vi "intake-shooter.vi"() -> ()   [LabVIEW 2023]
uses:
  ctrl defs/ctrl shooter speeds.ctl
  ctrl defs/ctrl intake speeds.ctl
  ctrl defs/ctrl INTAKE STATES.ctl
  ctrl defs/ctrl SHOOTER STATES.ctl
  <vilib>/Rock Robotics/WPI/MotorControl/WPI_MotorControlDeviceRef.ctl
  <vilib>/Rock Robotics/WPI/MotorControl/WPI_MotorControlType.ctl
  <vilib>/Rock Robotics/SystemInterfaces/DIO/FPGA_DIOPWMChannel.ctl
  <vilib>/Rock Robotics/WPI/PWM/WPI_PWMDeadband.ctl
  <vilib>/Rock Robotics/SystemInterfaces/DIO/FPGA_DIOChannel.ctl
  <vilib>/Rock Robotics/WPI/ThirdParty/REV Robotics/REVLib/Typedef/Spark MAX Control Type.ctl
  Global INIT.vi
  Global stack names.vi
  <vilib>/Rock Robotics/Network Tables/NT Read Boolean.vi
  <vilib>/Rock Robotics/Network Tables/NT Write String.vi
  <vilib>/Rock Robotics/Network Tables/NT Write Boolean.vi
panel:
  out "OVERIDE\nNOTE\nCHECK":bool
  in  "LOADER\nshoot\n%VBus":dbl
  in  "LOADER\nFeed Forward":dbl
  out "SHOOTER\ntarget %VBus":dbl=0.08
  out "Sensor Velocity":dbl=417.1380920410156
  out "SHOOTER\ntarget rpm":dbl=454.08
  out "SHOOTER\nVelocity (rpm)":dbl=417.1380920410156
  in  "AUTO run\nINTAKE after\nSHOT":bool
  in  "WRITE to global":bool
  in  "reload global values":bool
  in  "LOADER speeds":T1={"forward"=0.85, "reverse"=-1.0} {"reverse" min=-1.0 max=-0.02 format="%.3f"; "forward" min=0.02 max=1.0 format="%.3f"}
  in  "LOADER max/min":T1={"forward"=1.0, "reverse"=-1.0} {"reverse" min=-1.0 max=-0.02 format="%.3f"; "forward" min=0.02 max=1.0 format="%.3f"}
  in  "INTAKE speeds":T1={"forward"=1.0, "reverse"=-1.0} {"reverse" min=-1.0 max=-0.02 format="%.3f"; "forward" min=0.02 max=1.0 format="%.3f"}
  in  "SHOOTER speeds":T2={"SPEAKER"=1.0, "AMP"=0.08} {"AMP" min=0.02 max=1.0 format="%.3f"; "SPEAKER" min=0.02 max=1.0 format="%.3f"}
  in  "milliseconds to wait\nREV LOADER":u32=500
  in  "delay after\nSHOOT\ncommit (ms)":u32=500
  in  "delay for\nSPIN UP (ms)":u32=250
  in  "DISABLE\nNOTE CHECK for\nSHOOTING":bool=TRUE
  out "LOOKING\nfor NOTE":bool
  out "note sensor":bool
  in  "SHOOT STATUS":string="STANDBY"
  out "max rpm\n- SHOOTER":dbl=5676.0
  out "FIRE!":bool
  in  "INTAKE STATUS":string="Standby"
  out "max rpm\n- INTAKE":dbl=1419.0
  out "NOTE is\nloaded":bool
  out "run reverse":bool
  out "run intake":bool
  out "run? is\nACTIVE":bool
  in  "milliseconds to wait\nIN REVERSE":u32=1000
  in  "milliseconds to wait\nafter NOTE trigger":u32=100
  out "EXT FLAP":bool
  out "AMP OPT":bool
  in  "REVS to\nRETRACT":dbl=0.75 format="%#_13g"
  out "max rpm\n- LOADER":dbl=2750.0
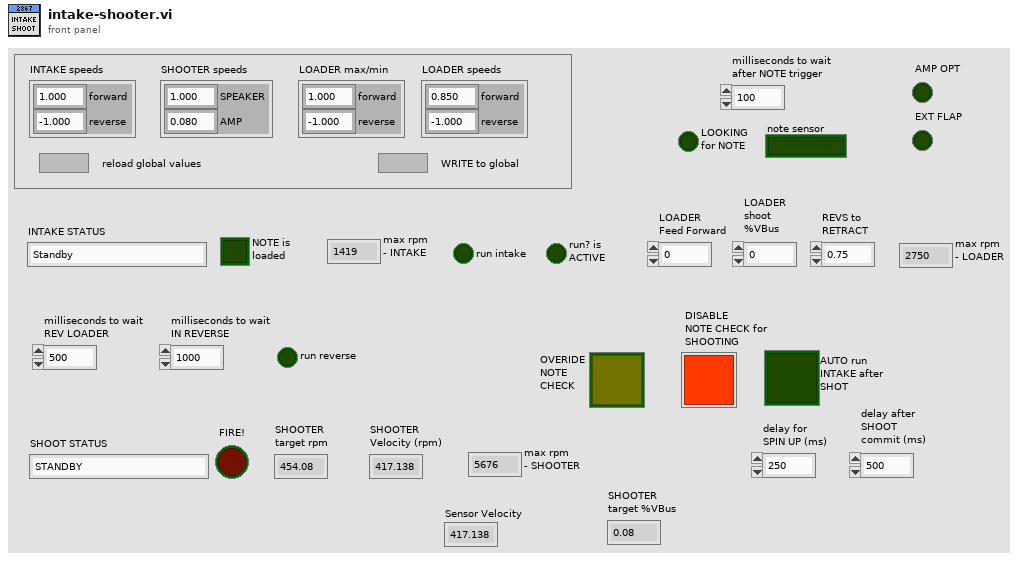
[diagram p1: front panel]
types:
  T1 = typedef "ctrl intake speeds.ctl" = cluster{"forward":dbl, "reverse":dbl}
  T2 = typedef "ctrl shooter speeds.ctl" = cluster{"SPEAKER":dbl, "AMP":dbl}
  T3 = typedef "ctrl SHOOTER STATES.ctl" = enum16{"STANDBY", "RETRACT NOTE", "SPIN-UP", "SHOOT", "RESET"}
  T4 = typedef "ctrl INTAKE STATES.ctl" = enum16{"STANDBY", "START INTAKES", "WATCH for NOTE", "SHUT DOWN", "REVERSE"}
  T5 = typedef "WPI_MotorControlDeviceRef.ctl" = cluster{"DeviceStatus":errorcluster, "Type":T6, "PWM":cluster{"PWM Channel":T7, "DeadBand":T8}, "CAN":cluster{"Device Number":u8, "SetOutput VI Ref":variant, "GetOutput VI Ref":variant, "Enable VI Ref":variant, "Disable VI Ref":variant, "Data":variant}, "Invert":bool, "DIO PWM":cluster{"PWM \"Enable\" Channel":T7, "DIOChannel":T9, "PWM Rate":dbl}}
  T6 = typedef "WPI_MotorControlType.ctl" = enum16{"PWM", "CAN", "DIO PWM"}
  T7 = typedef "FPGA_DIOPWMChannel.ctl" = enum8{"PWM 0", "PWM 1", "PWM 2", "PWM 3", "PWM 4", "PWM 5", "PWM 6", "PWM 7", "PWM 8", "PWM 9", "PWM MXP 0", "PWM MXP 1", "PWM MXP 2", "PWM MXP 3", "PWM MXP 4", "PWM MXP 5", "PWM MXP 6", "PWM MXP 7", "PWM MXP 8", "PWM MXP 9", "Invalid"}
  T8 = typedef "WPI_PWMDeadband.ctl" = cluster{"Name":string, "maxPositivePwm":i32, "minPositivePwm":i32, "centerPwm":i32, "maxNegativePwm":i32, "minNegativePwm":i32, "angularRange":u16}
  T9 = typedef "FPGA_DIOChannel.ctl" = enum8{"DIO 0", "DIO 1", "DIO 2", "DIO 3", "DIO 4", "DIO 5", "DIO 6", "DIO 7", "DIO 8", "DIO 9", "DIO MXP 0", "DIO MXP 1", "DIO MXP 2", "DIO MXP 3", "DIO MXP 4", "DIO MXP 5", "DIO MXP 6", "DIO MXP 7", "DIO MXP 8", "DIO MXP 9", "DIO MXP 10", "DIO MXP 11", "DIO MXP 12", "DIO MXP 13", "DIO MXP 14", "DIO MXP 15", "SPI Port CS1", "SPI Port CS2", "SPI Port CS3", "SPI Port MISO", "SPI Port MOSI", "Invalid"}
  T10 = cluster{"INTAKE ref":T5, "LOADER ref":T5, "SHOOTER ref":T5}
  T11 = typedef "ctrl DIO.ctl" = cluster{"description":string, "Installed?":bool, "DIOChannel":T9, "refnum name":string}
  T12 = typedef "ctrl swerve motor.ctl" = cluster{"description":string, "MOTOR SELECT":T13, "Installed?":bool, "CAN ID":u8, "refnum name":string, "Invert":bool, "Idle Mode":T14, "Current limiting":T15, "MOTOR PIDF coefficients":T16, "gear ratio":dbl}
  T13 = typedef "ctrl MOTOR SELECT.ctl" = i16
  T14 = typedef "Spark MAX Idle Mode.ctl" = enum16{"Coast", "Brake"}
  T15 = typedef "ctrl Spark MAX current limiting.ctl" = cluster{"Linearized":bool, "Free Speed (A)":dbl, "Primay (A)":dbl, "Limit RPM (0)":u32}
  T16 = typedef "ctrl motor PIDF coefficients.ctl" = cluster{"PIDF":cluster{"P Gain":dbl, "I Gain":dbl, "D Gain":dbl, "F Gain":dbl, "I Zone":dbl, "Min Output":dbl, "Max Output":dbl}, "Smart Motion":T17}
  T17 = typedef "Spark MAX Smart Motion Parameters.ctl" = cluster{"Max Velocity":dbl, "Max Acceleration":dbl, "Minimum Velocity Output":dbl, "Allowed Closed Loop Error":dbl}
  T18 = typedef "WPI_DigitalInputDevRef.ctl" = cluster{"DevStatus":errorcluster, "DIO Channel":T9}
  T19 = typedef "ctrl stack - INTAKE SHOOTER.ctl" = cluster{"INTAKE STATE":string, "RUN INTAKE?":string, "RUN REVERSE?":string, "NOTE LOADED?":string, "SHOOTER STATE":string, "SHOOTER FIRE?":string, "SHOOT AMP?":string, "EXTEND FLAP?":string, "LOOKING for NOTE":string, "OVERIDE NOTE CHECK":string}
  T20 = typedef "Spark MAX Control Type.ctl" = enum16{"Percent VBus", "Voltage", "Velocity", "Position", "Smart Motion", "Current", "Smart Velocity"}
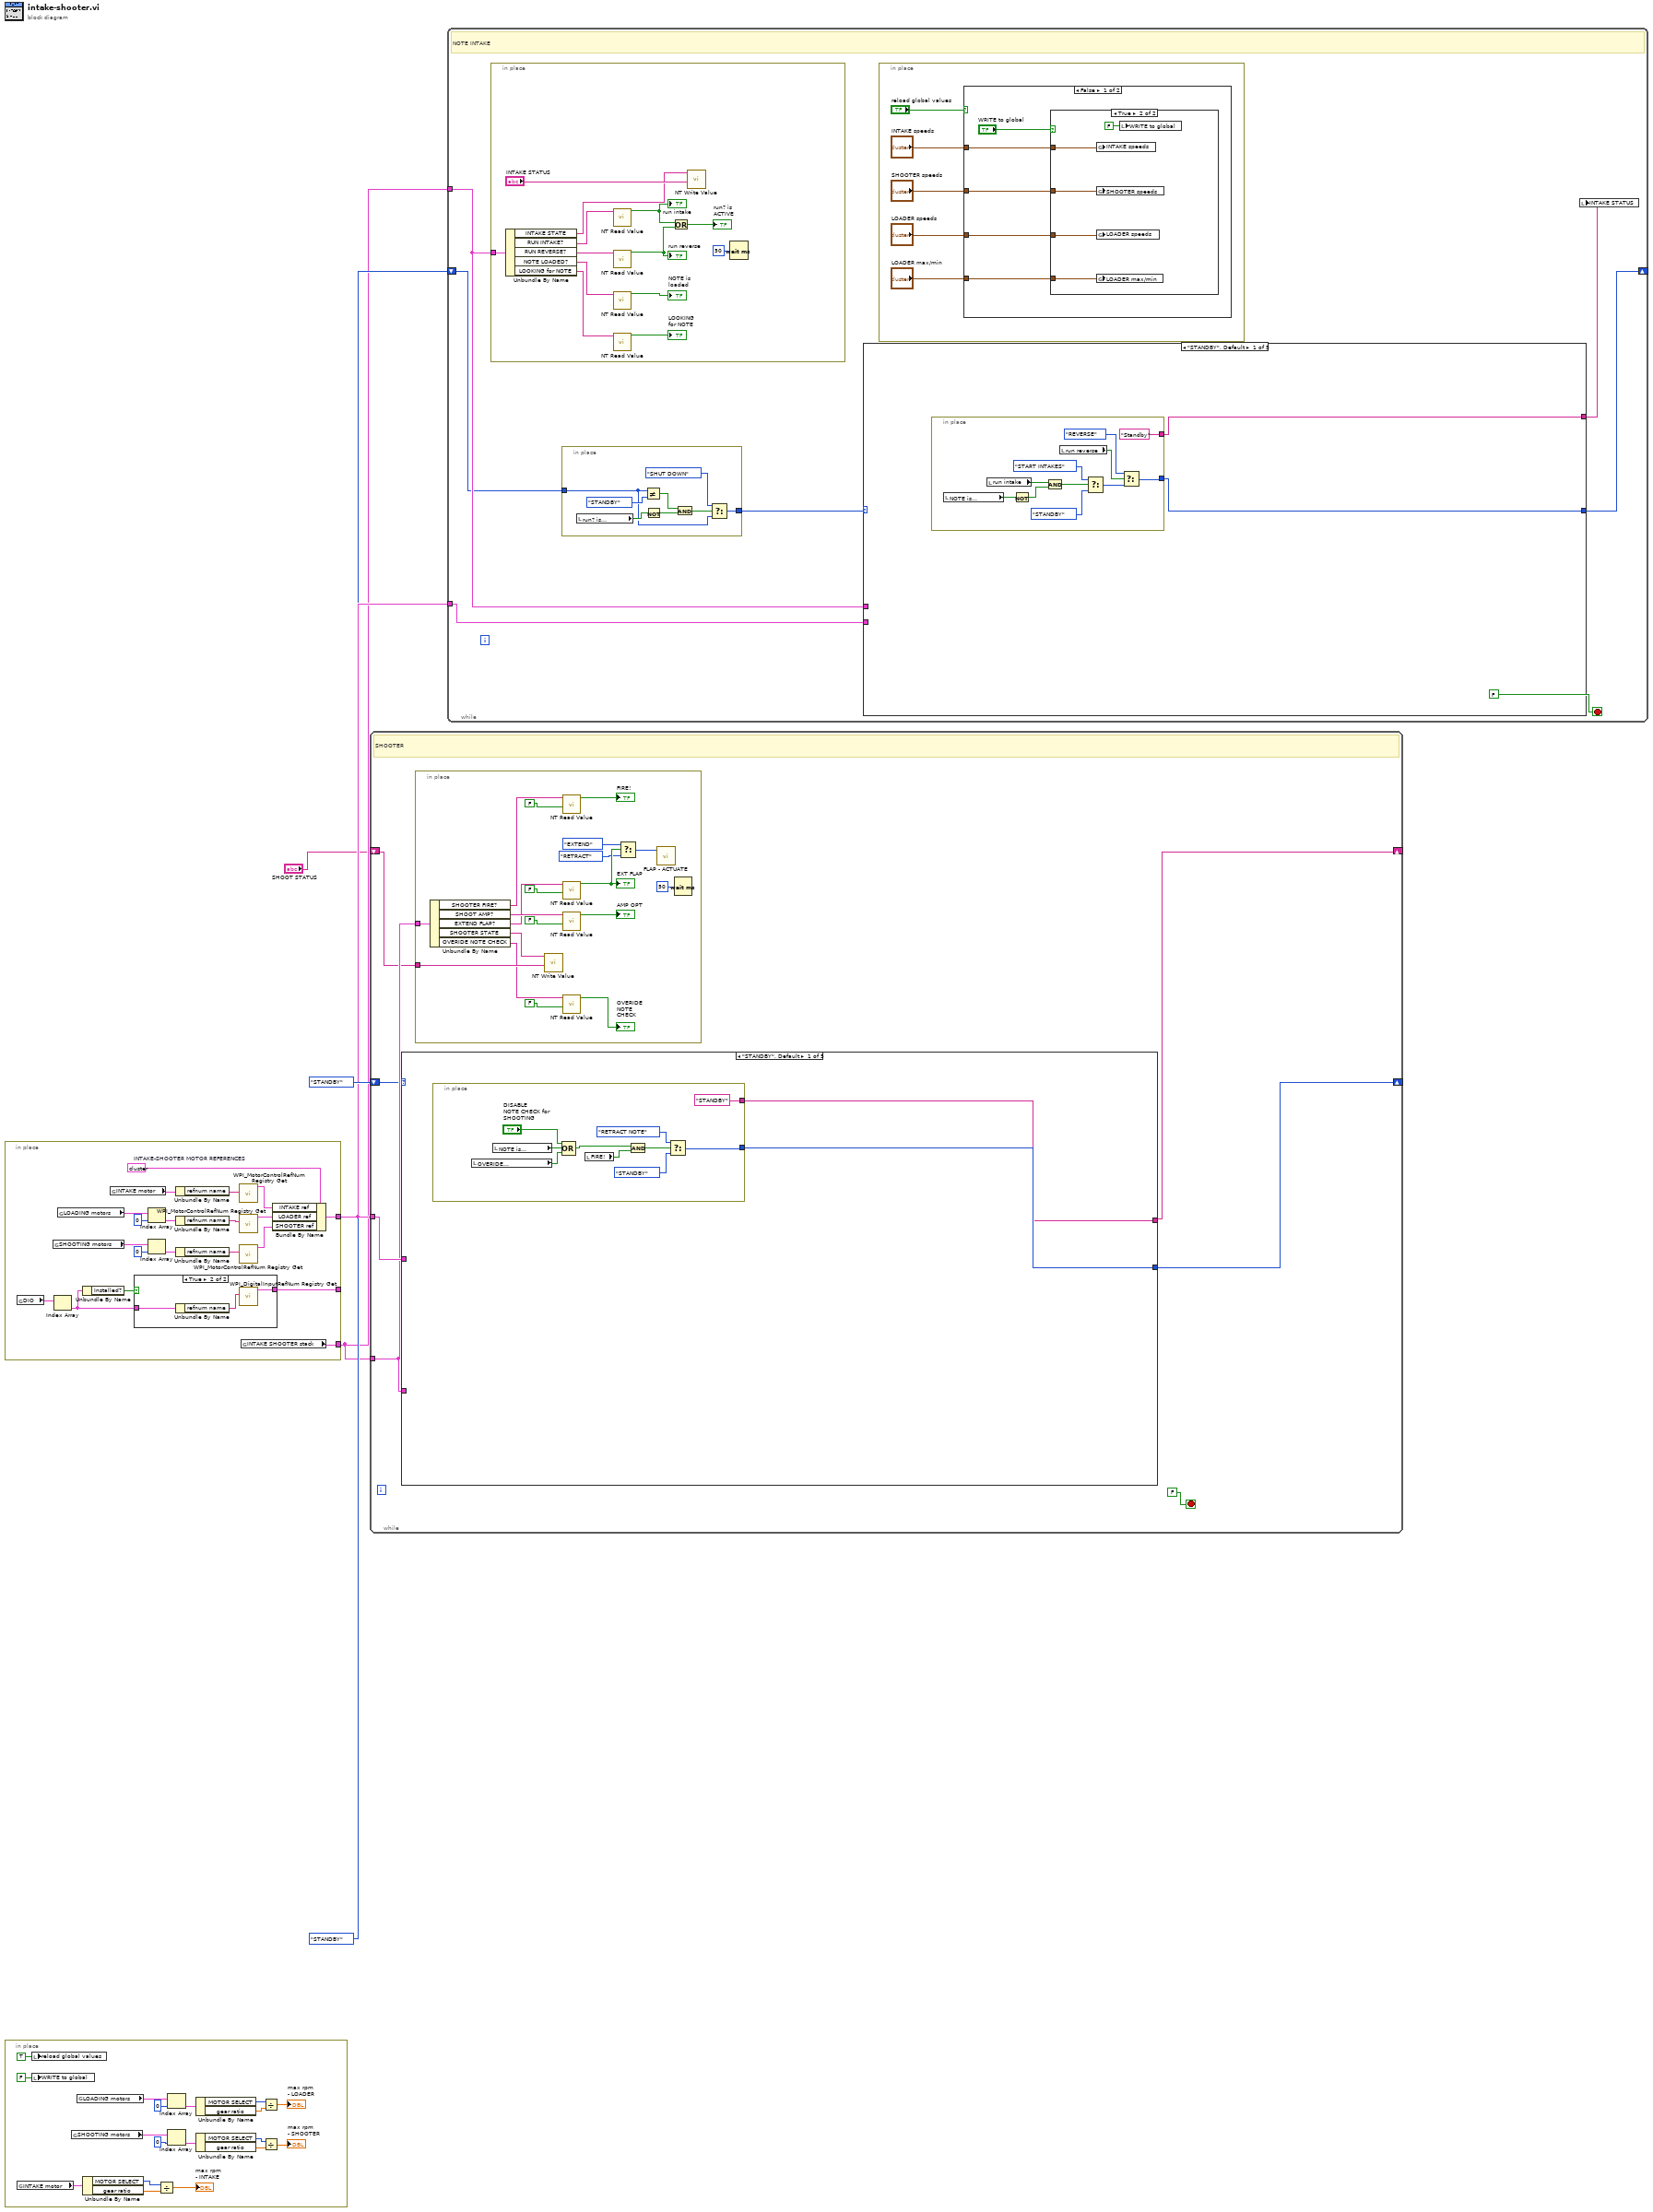
[diagram p0: block diagram]
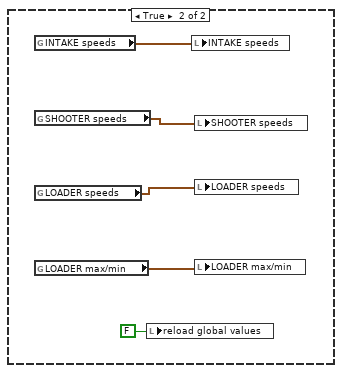
[diagram p3: hidden frame]
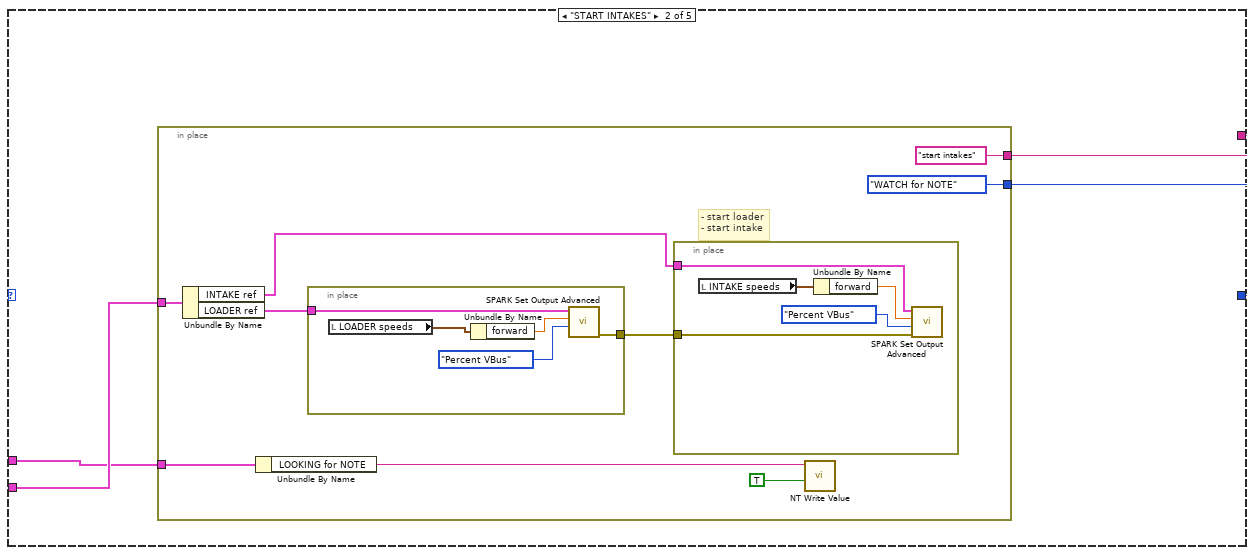
[diagram p4: hidden frame]
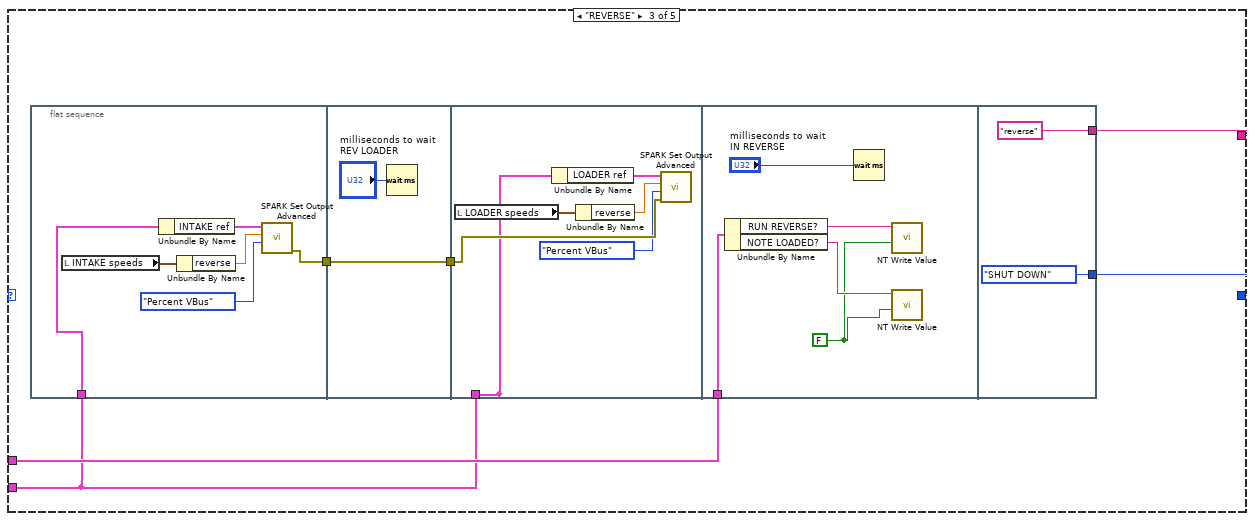
[diagram p5: hidden frame]
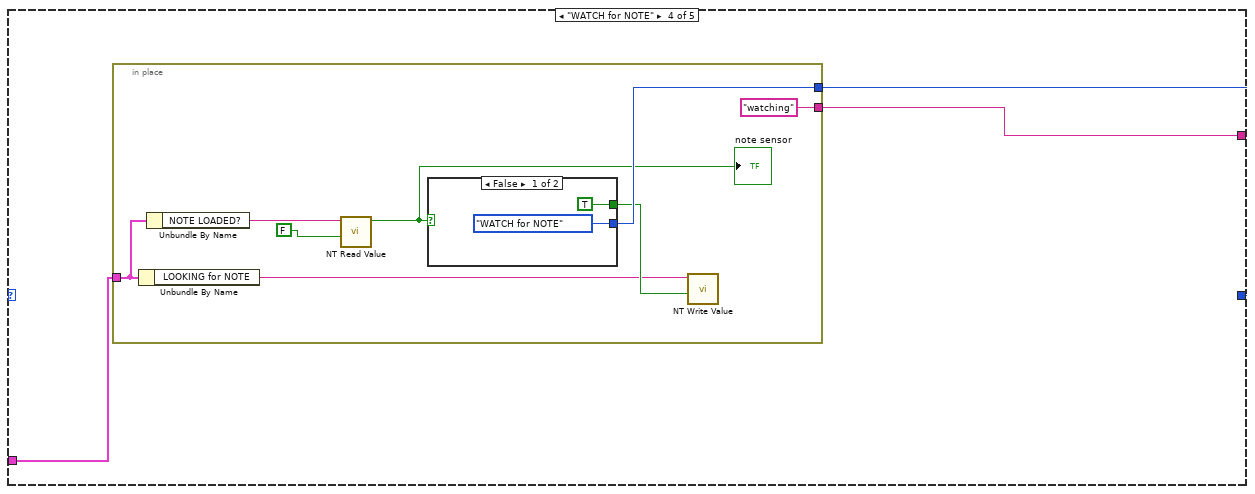
[diagram p6: hidden frame]
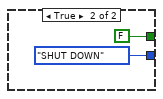
[diagram p7: hidden frame]
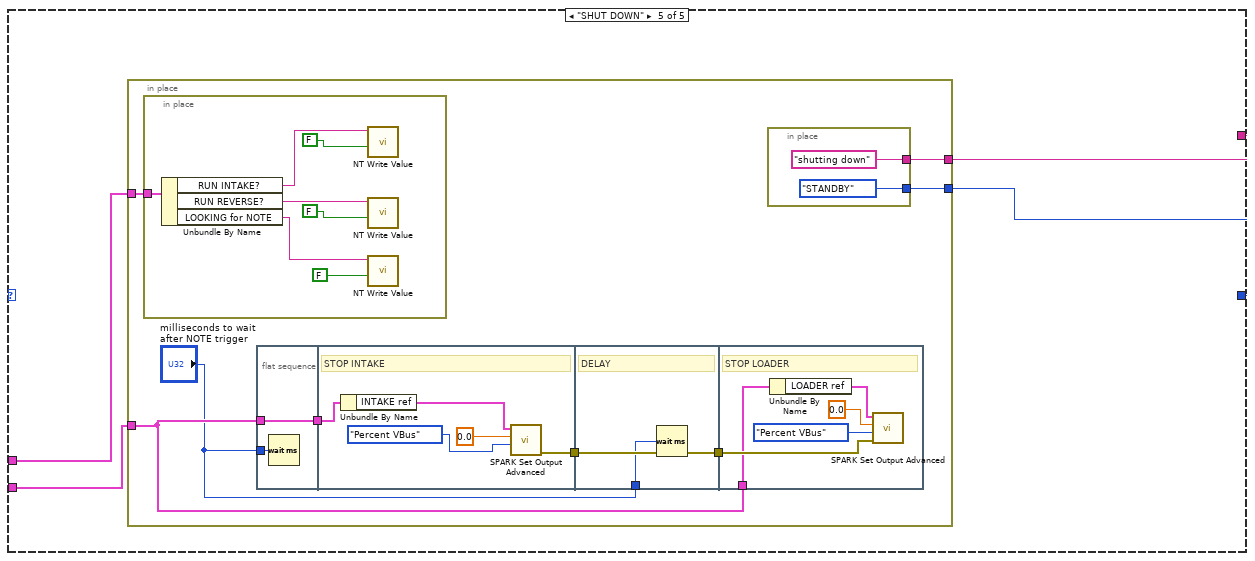
[diagram p8: hidden frame]
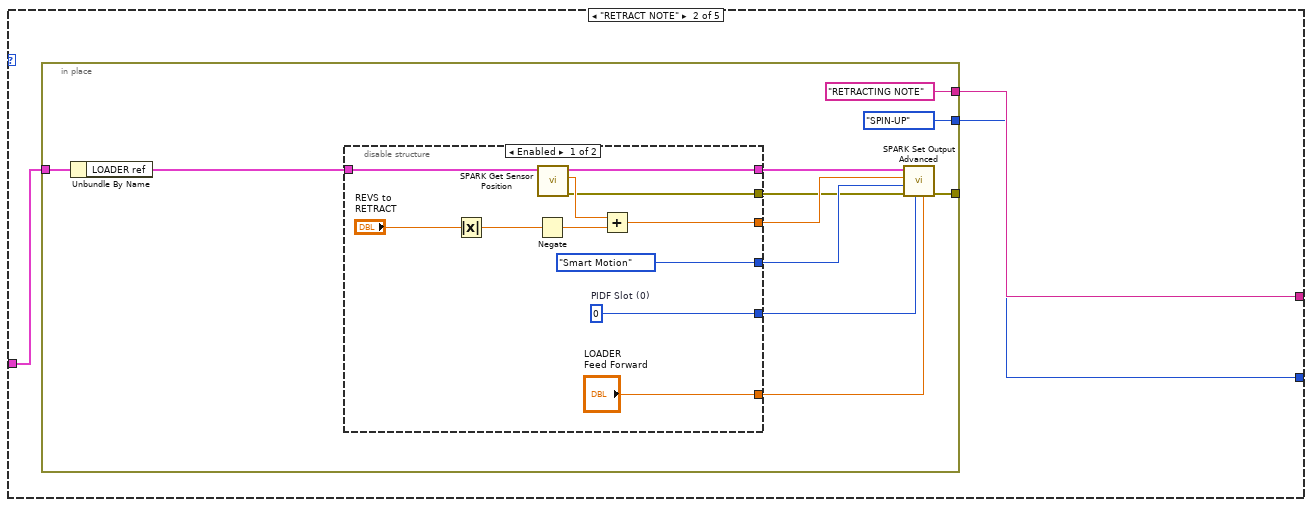
[diagram p9: hidden frame]
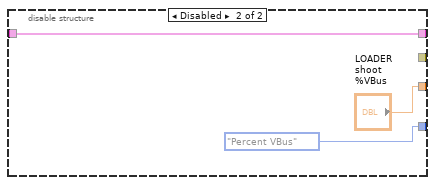
[diagram p10: hidden frame]
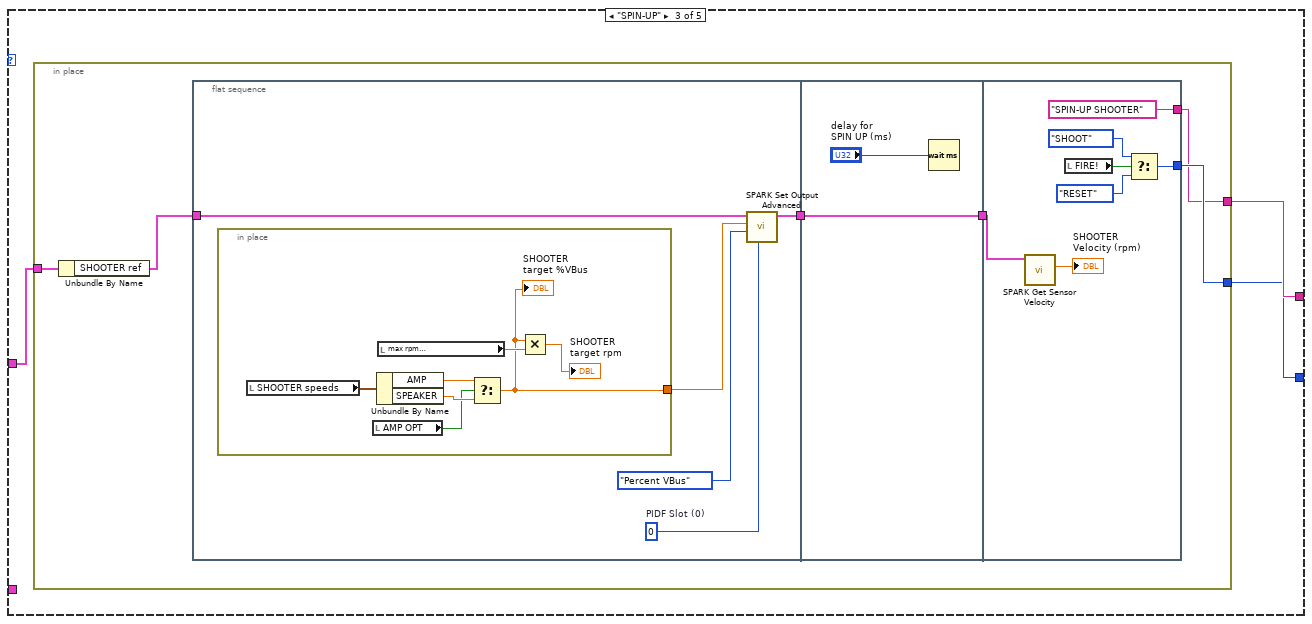
[diagram p11: hidden frame]
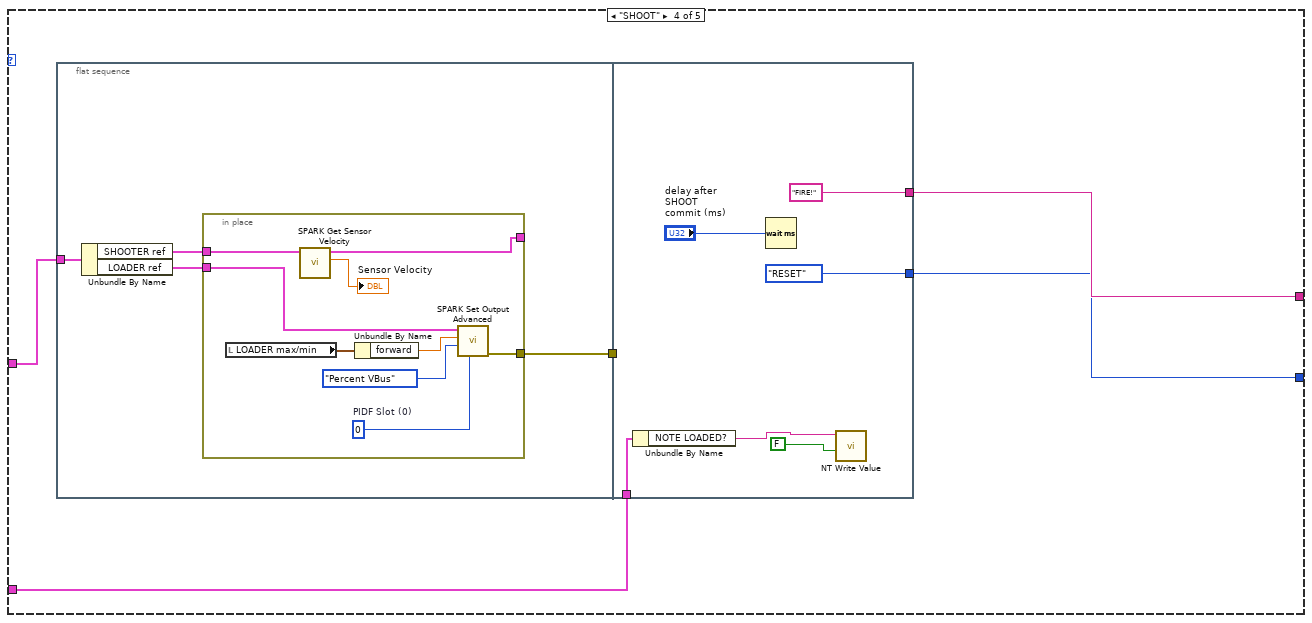
[diagram p12: hidden frame]
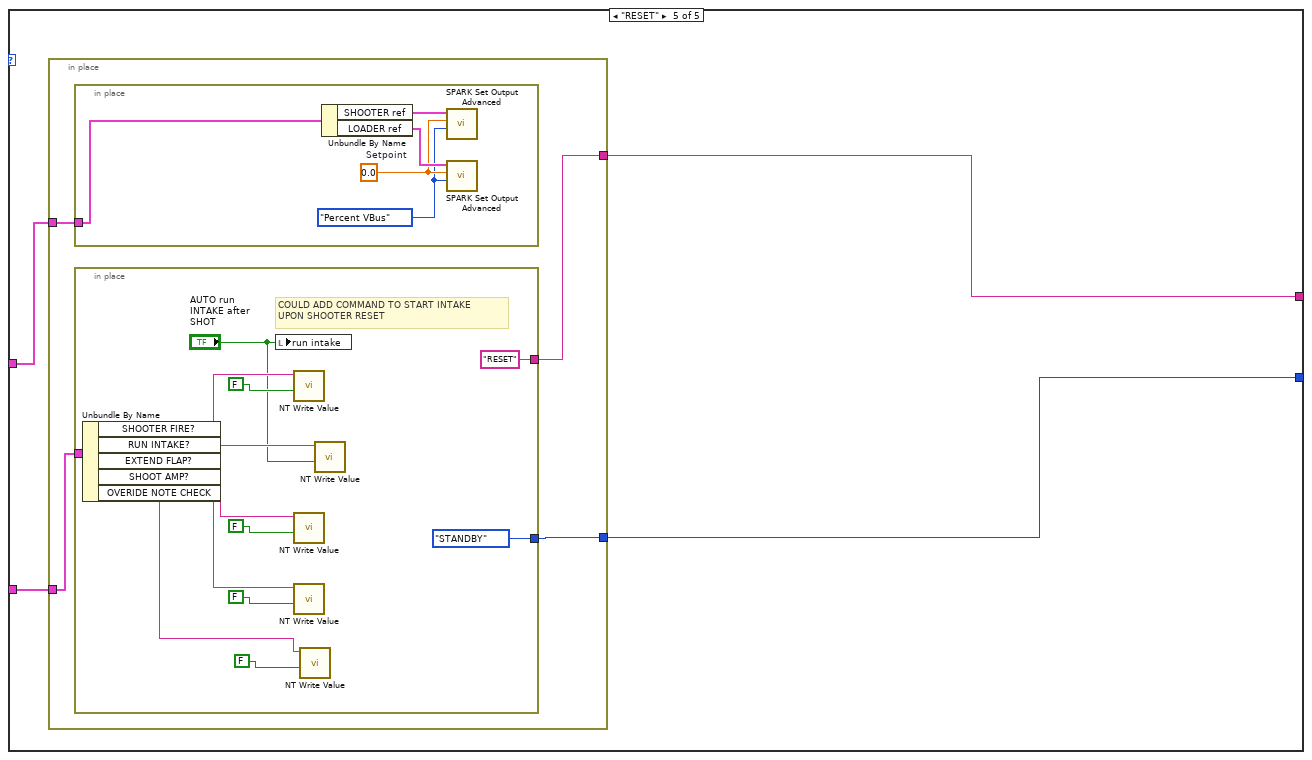
[diagram p13: hidden frame]
diagram:
  n1 = in-place {
    in-place-border: [w22] -> _
    in-place-border: [w7] -> w4
    in-place-border: [w6] -> w2
    w11 = T10 {"INTAKE ref"={"DeviceStatus"={"status"=FALSE, "code"=0, "source"=""}, "Type"=enum."PWM", "PWM"={"PWM Channel"=enum."Invalid", "DeadBand"={"Name"="", "maxPositivePwm"=0, "minPositivePwm"=0, "centerPwm"=0, "maxNegativePwm"=0, "minNegativePwm"=0, "angularRange"=0}}, "CAN"={"Device Number"=0, "SetOutput VI Ref"=variant(refnum<vi> refnum), "GetOutput VI Ref"=variant(refnum<vi> refnum), "Enable VI Ref"=variant(refnum<vi> refnum), "Disable VI Ref"=variant(refnum<vi> refnum), "Data"=variant}, "Invert"=FALSE, "DIO PWM"={"PWM \"Enable\" Channel"=enum."Invalid", "DIOChannel"=enum."Invalid", "PWM Rate"=0.0}}, "LOADER ref"={"DeviceStatus"={"status"=FALSE, "code"=0, "source"=""}, "Type"=enum."PWM", "PWM"={"PWM Channel"=enum."Invalid", "DeadBand"={"Name"="", "maxPositivePwm"=0, "minPositivePwm"=0, "centerPwm"=0, "maxNegativePwm"=0, "minNegativePwm"=0, "angularRange"=0}}, "CAN"={"Device Number"=0, "SetOutput VI Ref"=variant(refnum<vi> refnum), "GetOutput VI Ref"=variant(refnum<vi> refnum), "Enable VI Ref"=variant(refnum<vi> refnum), "Disable VI Ref"=variant(refnum<vi> refnum), "Data"=variant}, "Invert"=FALSE, "DIO PWM"={"PWM \"Enable\" Channel"=enum."Invalid", "DIOChannel"=enum."Invalid", "PWM Rate"=0.0}}, "SHOOTER ref"={"DeviceStatus"={"status"=FALSE, "code"=0, "source"=""}, "Type"=enum."PWM", "PWM"={"PWM Channel"=enum."Invalid", "DeadBand"={"Name"="", "maxPositivePwm"=0, "minPositivePwm"=0, "centerPwm"=0, "maxNegativePwm"=0, "minNegativePwm"=0, "angularRange"=0}}, "CAN"={"Device Number"=0, "SetOutput VI Ref"=variant(refnum<vi> refnum), "GetOutput VI Ref"=variant(refnum<vi> refnum), "Enable VI Ref"=variant(refnum<vi> refnum), "Disable VI Ref"=variant(refnum<vi> refnum), "Data"=variant}, "Invert"=FALSE, "DIO PWM"={"PWM \"Enable\" Channel"=enum."Invalid", "DIOChannel"=enum."Invalid", "PWM Rate"=0.0}}}  # INTAKE-SHOOTER MOTOR REFERENCES
    n2 = global read "Global INIT.vi" "DIO"() -> (w25:T11[])
    n3 = global read "Global INIT.vi" "SHOOTING motors"() -> (w20:T12[])
    n4 = Index Array(array=w25) -> (element=w23:T11)  [unwired: 1 in]
    n5 = global read "Global INIT.vi" "LOADING motors"() -> (w21:T12[])
    n6 = Unbundle By Name(w23) -> ("Installed?"=w24:bool)
    n7 = global read "Global INIT.vi" "INTAKE motor"() -> (w13:T12)
    n8 = case shown="True" w24 {
      tunnel: [_ w28] -> w22
      tunnel: w23 -> [_ w27]
      frame False {
      }
      frame True {
        n9 = Unbundle By Name(w27) -> ("refnum name"=w26:string)
        n10 = call <vilib>:"WPI_DigitalInputRefNum Registry Get.vi"("refnum name"=w26) -> ("DigitalInputDevRef"=w28:T18)  [unwired: 9 in, 1 out]
      }
    }
    n11 = Index Array(array=w21, index=0) -> (element=w17:T12)
    n12 = Index Array(array=w20, index=0) -> (element=w15:T12)
    n13 = Unbundle By Name(w13) -> ("refnum name"=w12:string)
    n14 = Unbundle By Name(w17) -> ("refnum name"=w16:string)
    n15 = Unbundle By Name(w15) -> ("refnum name"=w14:string)
    n16 = call <vilib>:"WPI_MotorControlRefNum Registry Get.vi"("refnum name"=w12) -> ("MotorControlDevRef"=w8:T5)  [unwired: 9 in, 1 out]
    n17 = call <vilib>:"WPI_MotorControlRefNum Registry Get.vi"("refnum name"=w16) -> ("MotorControlDevRef"=w9:T5)  [unwired: 9 in, 1 out]
    n18 = call <vilib>:"WPI_MotorControlRefNum Registry Get.vi"("refnum name"=w14) -> ("MotorControlDevRef"=w10:T5)  [unwired: 9 in, 1 out]
    n19 = global read "Global stack names.vi" "INTAKE SHOOTER stack"() -> (w6:T19)
    n20 = Bundle By Name(cluster=w11, "INTAKE ref"=w8, "LOADER ref"=w9, "SHOOTER ref"=w10) -> (w7:T10)
  }
  n21 = in-place {
    n22 = global read "Global INIT.vi" "INTAKE motor"() -> (w31:T12)
    n23 = local write "reload global values"(TRUE ("reload global values")) -> ()
    n24 = local write "WRITE to global"(FALSE ("WRITE to global")) -> ()
    n25 = global read "Global INIT.vi" "SHOOTING motors"() -> (w38:T12[])
    n26 = global read "Global INIT.vi" "LOADING motors"() -> (w43:T12[])
    n27 = Unbundle By Name(w31) -> ("MOTOR SELECT"=w33:T13, "gear ratio"=w32:dbl)
    n28 = Divide(x=w33, y=w32) -> (x/y=→"max rpm\n- INTAKE":dbl)
    n29 = Index Array(array=w43, index=0) -> (element=w41:T12)
    n30 = Index Array(array=w38, index=0) -> (element=w36:T12)
    n31 = Unbundle By Name(w41) -> ("MOTOR SELECT"=w40:T13, "gear ratio"=w39:dbl)
    n32 = Unbundle By Name(w36) -> ("MOTOR SELECT"=w35:T13, "gear ratio"=w34:dbl)
    n33 = Divide(x=w40, y=w39) -> (x/y=→"max rpm\n- LOADER":dbl)
    n34 = Divide(x=w35, y=w34) -> (x/y=→"max rpm\n- SHOOTER":dbl)
  }
  n35 = while {
    tunnel: w4 -> [w52]
    shift-right: [w53] -> _
    shift-left: ctrl_SHOOTER_STATES."STANDBY" -> [w49]
    tunnel: w2 -> [w50]
    shift-right: [w47] -> _
    shift-left: "SHOOT STATUS" -> [w48]
    stop <- FALSE stop-if-true
    # "SHOOTER"
    n36 = case shown="\"STANDBY\", Default" w49 {
      tunnel: [w55 w67 w94 w126 w149] -> w53
      tunnel: w52 -> [_ w66 w96 w128 w151]
      tunnel: [w54 w68 w95 w127 w150] -> w47
      tunnel: w50 -> [_ _ _ w124 w148]
      frame "STANDBY", Default {
        n37 = in-place {
          in-place-border: [w64] -> w55
          in-place-border: ["STANDBY" ("value")] -> w54
          n38 = local read "OVERIDE\nNOTE\nCHECK"() -> (w56:bool)
          n39 = local read "NOTE is\nloaded"() -> (w58:bool)
          n40 = Compound Arithmetic op=OR("DISABLE\nNOTE CHECK for\nSHOOTING", w58, w56) -> (w57:bool)
          n41 = local read "FIRE!"() -> (w62:bool)
          n42 = And(x=w57, y=w62) -> (x .and. y?=w63:bool)
          n43 = Select(t=ctrl_SHOOTER_STATES."RETRACT NOTE", s=w63, f=ctrl_SHOOTER_STATES."STANDBY") -> (s? t:f=w64:T3)
        }
      }
      frame "RETRACT NOTE" {
        n44 = in-place {
          in-place-border: ["RETRACTING NOTE" ("value")] -> w68
          in-place-border: [ctrl_SHOOTER_STATES."SPIN-UP"] -> w67
          in-place-border: [w73] -> _
          in-place-border: w66 -> [w72]
          n45 = Unbundle By Name(w72) -> ("LOADER ref"=w71:T5)
          n46 = disable-structure shown="Enabled" {
            disable-tunnel: [Spark_MAX_Control_Type."Smart Motion" ("Control Mode") Spark_MAX_Control_Type."Percent VBus" ("Control Mode")] -> w77
            disable-tunnel: [w89 _] -> w76
            disable-tunnel: [w88 w93] -> w75
            disable-tunnel: [w87 "LOADER\nshoot\n%VBus"] -> w74
            disable-tunnel: w71 -> [w85 w93]
            disable-tunnel: ["LOADER\nFeed Forward" _] -> w70
            disable-tunnel: [w80 _] -> w69
            frame Enabled {
              w89 = 0  # PIDF Slot (0)
              n47 = Absolute Value(x="REVS to\nRETRACT") -> (abs(x)=w83:dbl)
              n48 = Negate(x=w83) -> (-x=w82:dbl)
              n49 = call <vilib>:"SPARK Get Sensor Position.vi"("MotorControlDevRef in"=w85) -> ("error out"=w80:errorcluster, "Sensor Position"=w86:dbl, "MotorControlDevRef out"=w88:T5)  [unwired: 7 in, 1 out]
              n50 = Add(x=w86, y=w82) -> (x+y=w87:dbl)
            }
            frame Disabled {
            }
          }
          n51 = call <vilib>:"SPARK Set Output Advanced.vi"("Arbitrary Feed Forward (0)"=w70, "PIDF Slot (0)"=w76, "error in (no error)"=w69, "Control Mode"=w77, "Setpoint"=w74, "MotorControlDevRef"=w75) -> ("error out"=w73:errorcluster)  [unwired: 4 in, 1 out]
        }
      }
      frame "SPIN-UP" {
        n52 = in-place {
          in-place-border: w96 -> [w102]
          in-place-border: [w99] -> w95
          in-place-border: [w100] -> w94
          n53 = Unbundle By Name(w102) -> ("SHOOTER ref"=w101:T5)
          n54 = flat-sequence {
            tunnel: w101 -> [w107]
            tunnel: [w104] -> w98
            tunnel: w98 -> [w115]
            tunnel: [w115] -> w97
            tunnel: [w121] -> w100
            tunnel: ["SPIN-UP SHOOTER" ("value")] -> w99
            tunnel: w97 -> [w117]
            frame #0 {
              w105 = 0  # PIDF Slot (0)
              n55 = in-place {
                in-place-border: [w108] -> w103
                n56 = local read "SHOOTER speeds"() -> (w111:T2)
                n57 = local read "AMP OPT"() -> (w112:bool)
                n58 = Unbundle By Name(w111) -> ("AMP"=w113:dbl, "SPEAKER"=w114:dbl)
                n59 = local read "max rpm\n- SHOOTER"() -> (w109:dbl)
                n60 = Select(t=w113, s=w112, f=w114) -> (s? t:f=w108:dbl)
                "SHOOTER\ntarget %VBus" <- w108
                n61 = Multiply(x=w108, y=w109) -> (x*y=→"SHOOTER\ntarget rpm":dbl)
              }
              n62 = call <vilib>:"SPARK Set Output Advanced.vi"("PIDF Slot (0)"=w105, "Control Mode"=Spark_MAX_Control_Type."Percent VBus", "Setpoint"=w103, "MotorControlDevRef"=w107) -> ("MotorControlDevRef"=w104:T5)  [unwired: 6 in, 1 out]
            }
            frame #1 {
              n63 = Wait (ms)(milliseconds to wait="delay for\nSPIN UP (ms)") -> ()  [unwired: 1 out]
            }
            frame #2 {
              n64 = call <vilib>:"SPARK Get Sensor Velocity.vi"("MotorControlDevRef in"=w117) -> ("Sensor Velocity"=→"SHOOTER\nVelocity (rpm)":dbl)  [unwired: 7 in, 3 out]
              n65 = local read "FIRE!"() -> (w123:bool)
              n66 = Select(t=ctrl_SHOOTER_STATES."SHOOT", s=w123, f=ctrl_SHOOTER_STATES."RESET") -> (s? t:f=w121:T3)
            }
          }
        }
      }
      frame "SHOOT" {
        n67 = flat-sequence {
          tunnel: w128 -> [w132]
          tunnel: [w129] -> w125
          tunnel: ["FIRE!" ("value")] -> w127
          tunnel: [ctrl_SHOOTER_STATES."RESET"] -> w126
          tunnel: w125 -> [_]
          tunnel: w124 -> [w142]
          frame #0 {
            n68 = Unbundle By Name(w132) -> ("SHOOTER ref"=w130:T5, "LOADER ref"=w131:T5)
            n69 = in-place {
              in-place-border: w131 -> [w141]
              in-place-border: w130 -> [w136]
              in-place-border: [w135] -> _
              in-place-border: [w134] -> w129
              w140 = 0  # PIDF Slot (0)
              n70 = local read "LOADER max/min"() -> (w138:T1)
              n71 = call <vilib>:"SPARK Get Sensor Velocity.vi"("MotorControlDevRef in"=w136) -> ("Sensor Velocity"=→"Sensor Velocity":dbl, "MotorControlDevRef out"=w135:T5)  [unwired: 7 in, 2 out]
              n72 = Unbundle By Name(w138) -> ("forward"=w137:dbl)
              n73 = call <vilib>:"SPARK Set Output Advanced.vi"("PIDF Slot (0)"=w140, "Control Mode"=Spark_MAX_Control_Type."Percent VBus", "Setpoint"=w137, "MotorControlDevRef"=w141) -> ("error out"=w134:errorcluster)  [unwired: 6 in, 1 out]
            }
          }
          frame #1 {
            n74 = Unbundle By Name(w142) -> ("NOTE LOADED?"=w144:string)
            n75 = Wait (ms)(milliseconds to wait="delay after\nSHOOT\ncommit (ms)") -> ()  [unwired: 1 out]
            n76 = call-poly <vilib>:"NT Write Value.vi"("value"=FALSE, "name"=w144) -> ()  [unwired: 9 in, 1 out]
          }
        }
      }
      frame "RESET" {
        n77 = in-place {
          in-place-border: w151 -> [w155]
          in-place-border: [w152] -> w150
          in-place-border: [w153] -> w149
          in-place-border: w148 -> [w154]
          n78 = in-place {
            in-place-border: w155 -> [w158]
            w157 = 0.0  # Setpoint
            w156 = Spark_MAX_Control_Type."Percent VBus" ("Control Mode")
            n79 = Unbundle By Name(w158) -> ("SHOOTER ref"=w159:T5, "LOADER ref"=w160:T5)
            n80 = call <vilib>:"SPARK Set Output Advanced.vi"("Control Mode"=w156, "Setpoint"=w157, "MotorControlDevRef"=w159) -> ()  [unwired: 7 in, 2 out]
            n81 = call <vilib>:"SPARK Set Output Advanced.vi"("Control Mode"=w156, "Setpoint"=w157, "MotorControlDevRef"=w160) -> ()  [unwired: 7 in, 2 out]
          }
          n82 = in-place {
            in-place-border: w154 -> [w172]
            in-place-border: [ctrl_SHOOTER_STATES."STANDBY"] -> w153
            in-place-border: ["RESET" ("value")] -> w152
            # "COULD ADD COMMAND TO START INTAKE\nUPON SHOOTER RESET"
            n83 = Unbundle By Name(w172) -> ("SHOOTER FIRE?"=w171:string, "RUN INTAKE?"=w170:string, "EXTEND FLAP?"=w168:string, "SHOOT AMP?"=w165:string, "OVERIDE NOTE CHECK"=w161:string)
            n84 = local write "run intake"("AUTO run\nINTAKE after\nSHOT") -> ()
            n85 = call-poly <vilib>:"NT Write Value.vi"("value"=FALSE ("default value"), "name"=w171) -> ()  [unwired: 9 in, 1 out]
            n86 = call-poly <vilib>:"NT Write Value.vi"("value"=FALSE, "name"=w168) -> ()  [unwired: 9 in, 1 out]
            n87 = call-poly <vilib>:"NT Write Value.vi"("value"=FALSE, "name"=w165) -> ()  [unwired: 9 in, 1 out]
            n88 = call-poly <vilib>:"NT Write Value.vi"("value"=FALSE, "name"=w161) -> ()  [unwired: 9 in, 1 out]
            n89 = call-poly <vilib>:"NT Write Value.vi"("value"="AUTO run\nINTAKE after\nSHOT", "name"=w170) -> ()  [unwired: 9 in, 1 out]
          }
        }
      }
    }
    n90 = in-place {
      in-place-border: w50 -> [w191]
      in-place-border: w48 -> [w177]
      n91 = Unbundle By Name(w191) -> ("SHOOTER FIRE?"=w190:string, "SHOOT AMP?"=w188:string, "EXTEND FLAP?"=w185:string, "SHOOTER STATE"=w179:string, "OVERIDE NOTE CHECK"=w176:string)
      n92 = call-poly <vilib>:"NT Write Value.vi"("value"=w177, "name"=w179) -> ()  [unwired: 9 in, 1 out]
      n93 = call-poly <vilib>:"NT Read Value.vi"("default value"=FALSE, "name"=w190) -> ("value"=→"FIRE!":bool)  [unwired: 7 in, 2 out]
      n94 = call-poly <vilib>:"NT Read Value.vi"("default value"=FALSE, "name"=w185) -> ("value"=w182:bool)  [unwired: 7 in, 2 out]
      "EXT FLAP" <- w182
      n95 = call-poly <vilib>:"NT Read Value.vi"("default value"=FALSE, "name"=w188) -> ("value"=→"AMP OPT":bool)  [unwired: 7 in, 2 out]
      n96 = call-poly <vilib>:"NT Read Value.vi"("default value"=FALSE, "name"=w176) -> ("value"=→"OVERIDE\nNOTE\nCHECK":bool)  [unwired: 7 in, 2 out]
      n97 = Select(t=enum16{"EXTEND", "RETRACT"}."EXTEND" ("STATE"), s=w182, f=enum16{"EXTEND", "RETRACT"}."RETRACT" ("STATE")) -> (s? t:f=w184:enum16{"EXTEND", "RETRACT"})
      n98 = call "FLAP - ACTUATE.vi"("STATE"=w184) -> ()  [unwired: 10 in, 1 out]
      n99 = Wait (ms)(milliseconds to wait=u32 50) -> ()  [unwired: 1 out]
    }
  }
  n100 = while {
    shift-right: [w198] -> _
    shift-left: ctrl_INTAKE_STATES."STANDBY" ("INTAKE STATE") -> [w196]
    tunnel: w4 -> [w193]
    tunnel: w2 -> [w197]
    stop <- FALSE stop-if-true
    # "NOTE INTAKE"
    n101 = in-place {
      in-place-border: w197 -> [w349]
      n102 = Unbundle By Name(w349) -> ("INTAKE STATE"=w344:string, "RUN INTAKE?"=w351:string, "RUN REVERSE?"=w350:string, "NOTE LOADED?"=w352:string, "LOOKING for NOTE"=w341:string)
      n103 = call-poly <vilib>:"NT Read Value.vi"("name"=w351) -> ("value"=w348:bool)  [unwired: 8 in, 2 out]
      "run intake" <- w348
      n104 = call-poly <vilib>:"NT Read Value.vi"("name"=w350) -> ("value"=w347:bool)  [unwired: 8 in, 2 out]
      "run reverse" <- w347
      n105 = call-poly <vilib>:"NT Read Value.vi"("name"=w352) -> ("value"=→"NOTE is\nloaded":bool)  [unwired: 8 in, 2 out]
      n106 = call-poly <vilib>:"NT Read Value.vi"("name"=w341) -> ("value"=→"LOOKING\nfor NOTE":bool)  [unwired: 8 in, 2 out]
      n107 = Or(x=w348, y=w347) -> (x .or. y?=→"run? is\nACTIVE":bool)
      n108 = call-poly <vilib>:"NT Write Value.vi"("value"="INTAKE STATUS", "name"=w344) -> ()  [unwired: 9 in, 1 out]
      n109 = Wait (ms)(milliseconds to wait=u32 50) -> ()  [unwired: 1 out]
    }
    n110 = in-place {
      in-place-border: w196 -> [w220]
      in-place-border: [w223] -> w195
      n111 = local read "run? is\nACTIVE"() -> (w224:bool)
      n112 = Not Equal?(x=w220, y=ctrl_INTAKE_STATES."STANDBY" ("INTAKE STATE")) -> (x != y?=w227:bool)
      n113 = Not(x=w224) -> (.not. x?=w225:bool)
      n114 = And(x=w227, y=w225) -> (x .and. y?=w221:bool)
      n115 = Select(t=ctrl_INTAKE_STATES."SHUT DOWN" ("INTAKE STATE"), s=w221, f=w220) -> (s? t:f=w223:T4)
    }
    n116 = case shown="\"STANDBY\", Default" w195 {
      tunnel: [w229 w244 w268 w292 w309] -> w198
      tunnel: [w228 w243 w267 w293 w308] -> w194
      tunnel: w193 -> [_ w242 w264 _ w307]
      tunnel: w197 -> [_ w241 w269 w291 w306]
      frame "STANDBY", Default {
        n117 = in-place {
          in-place-border: [w235] -> w229
          in-place-border: ["Standby" ("value")] -> w228
          n118 = local read "NOTE is\nloaded"() -> (w232:bool)
          n119 = local read "run intake"() -> (w231:bool)
          n120 = Not(x=w232) -> (.not. x?=w238:bool)
          n121 = And(x=w231, y=w238) -> (x .and. y?=w239:bool)
          n122 = local read "run reverse"() -> (w233:bool)
          n123 = Select(t=ctrl_INTAKE_STATES."START INTAKES" ("INTAKE STATE 2"), s=w239, f=ctrl_INTAKE_STATES."STANDBY" ("INTAKE STATE 2")) -> (s? t:f=w236:T4)
          n124 = Select(t=ctrl_INTAKE_STATES."REVERSE" ("INTAKE STATE 2"), s=w233, f=w236) -> (s? t:f=w235:T4)
        }
      }
      frame "START INTAKES" {
        n125 = in-place {
          in-place-border: [ctrl_INTAKE_STATES."WATCH for NOTE" ("INTAKE STATE 2")] -> w244
          in-place-border: ["start intakes" ("value")] -> w243
          in-place-border: w242 -> [w251]
          in-place-border: w241 -> [w246]
          # "- start loader\n- start intake"
          n126 = Unbundle By Name(w251) -> ("INTAKE ref"=w250:T5, "LOADER ref"=w249:T5)
          n127 = Unbundle By Name(w246) -> ("LOOKING for NOTE"=w247:string)
          n128 = in-place {
            in-place-border: w249 -> [w258]
            in-place-border: [w256] -> w248
            n129 = local read "LOADER speeds"() -> (w254:T1)
            n130 = Unbundle By Name(w254) -> ("forward"=w255:dbl)
            n131 = call <vilib>:"SPARK Set Output Advanced.vi"("Control Mode"=Spark_MAX_Control_Type."Percent VBus", "Setpoint"=w255, "MotorControlDevRef"=w258) -> ("error out"=w256:errorcluster)  [unwired: 7 in, 1 out]
          }
          n132 = in-place {
            in-place-border: w250 -> [w263]
            in-place-border: w248 -> [w261]
            n133 = local read "INTAKE speeds"() -> (w260:T1)
            n134 = Unbundle By Name(w260) -> ("forward"=w259:dbl)
            n135 = call <vilib>:"SPARK Set Output Advanced.vi"("error in (no error)"=w261, "Control Mode"=Spark_MAX_Control_Type."Percent VBus", "Setpoint"=w259, "MotorControlDevRef"=w263) -> ()  [unwired: 6 in, 2 out]
          }
          n136 = call-poly <vilib>:"NT Write Value.vi"("value"=TRUE, "name"=w247) -> ()  [unwired: 9 in, 1 out]
        }
      }
      frame "REVERSE" {
        n137 = flat-sequence {
          tunnel: w264 -> [w273]
          tunnel: [w270] -> w266
          tunnel: w266 -> [w277]
          tunnel: [w277] -> w265
          tunnel: w265 -> [w283]
          tunnel: [w279] -> _
          tunnel: w264 -> [w279]
          tunnel: w269 -> [w287]
          tunnel: [ctrl_INTAKE_STATES."SHUT DOWN" ("INTAKE STATE 2")] -> w268
          tunnel: ["reverse" ("value")] -> w267
          frame #0 {
            n138 = local read "INTAKE speeds"() -> (w272:T1)
            n139 = Unbundle By Name(w273) -> ("INTAKE ref"=w275:T5)
            n140 = Unbundle By Name(w272) -> ("reverse"=w271:dbl)
            n141 = call <vilib>:"SPARK Set Output Advanced.vi"("Control Mode"=Spark_MAX_Control_Type."Percent VBus", "Setpoint"=w271, "MotorControlDevRef"=w275) -> ("error out"=w270:errorcluster)  [unwired: 7 in, 1 out]
          }
          frame #1 {
            n142 = Wait (ms)(milliseconds to wait="milliseconds to wait\nREV LOADER") -> ()  [unwired: 1 out]
          }
          frame #2 {
            n143 = local read "LOADER speeds"() -> (w282:T1)
            n144 = Unbundle By Name(w279) -> ("LOADER ref"=w278:T5)
            n145 = Unbundle By Name(w282) -> ("reverse"=w281:dbl)
            n146 = call <vilib>:"SPARK Set Output Advanced.vi"("error in (no error)"=w283, "Control Mode"=Spark_MAX_Control_Type."Percent VBus", "Setpoint"=w281, "MotorControlDevRef"=w278) -> ()  [unwired: 6 in, 2 out]
          }
          frame #3 {
            w285 = FALSE ("value")
            n147 = Unbundle By Name(w287) -> ("RUN REVERSE?"=w284:string, "NOTE LOADED?"=w288:string)
            n148 = Wait (ms)(milliseconds to wait="milliseconds to wait\nIN REVERSE") -> ()  [unwired: 1 out]
            n149 = call-poly <vilib>:"NT Write Value.vi"("value"=w285, "name"=w284) -> ()  [unwired: 9 in, 1 out]
            n150 = call-poly <vilib>:"NT Write Value.vi"("value"=w285, "name"=w288) -> ()  [unwired: 9 in, 1 out]
          }
          frame #4 {
          }
        }
      }
      frame "WATCH for NOTE" {
        n151 = in-place {
          in-place-border: ["watching" ("value")] -> w293
          in-place-border: [w300] -> w292
          in-place-border: w291 -> [w297]
          n152 = Unbundle By Name(w297) -> ("LOOKING for NOTE"=w294:string)
          n153 = Unbundle By Name(w297) -> ("NOTE LOADED?"=w298:string)
          n154 = call-poly <vilib>:"NT Read Value.vi"("default value"=FALSE ("value"), "name"=w298) -> ("value"=w296:bool)  [unwired: 7 in, 2 out]
          "note sensor" <- w296
          n155 = case shown="False" w296 {
            tunnel: [ctrl_INTAKE_STATES."WATCH for NOTE" ("INTAKE STATE 2") ctrl_INTAKE_STATES."SHUT DOWN" ("INTAKE STATE 2")] -> w300
            tunnel: [TRUE ("value") FALSE ("value")] -> w295
            frame False {
            }
            frame True {
            }
          }
          n156 = call-poly <vilib>:"NT Write Value.vi"("value"=w295, "name"=w294) -> ()  [unwired: 9 in, 1 out]
        }
      }
      frame "SHUT DOWN" {
        n157 = in-place {
          in-place-border: [w315] -> w309
          in-place-border: [w314] -> w308
          in-place-border: w307 -> [w313]
          in-place-border: w306 -> [w312]
          n158 = in-place {
            in-place-border: w312 -> [w338]
            n159 = Unbundle By Name(w338) -> ("RUN INTAKE?"=w337:string, "RUN REVERSE?"=w336:string, "LOOKING for NOTE"=w335:string)
            n160 = call-poly <vilib>:"NT Write Value.vi"("value"=FALSE, "name"=w337) -> ()  [unwired: 9 in, 1 out]
            n161 = call-poly <vilib>:"NT Write Value.vi"("value"=FALSE, "name"=w336) -> ()  [unwired: 9 in, 1 out]
            n162 = call-poly <vilib>:"NT Write Value.vi"("value"=FALSE, "name"=w335) -> ()  [unwired: 9 in, 1 out]
          }
          n163 = flat-sequence {
            tunnel: w313 -> [w319]
            tunnel: [w319] -> w311
            tunnel: "milliseconds to wait\nafter NOTE trigger" -> [w318]
            tunnel: [w324] -> w317
            tunnel: w311 -> [w323]
            tunnel: w317 -> [w326]
            tunnel: [w326] -> w316
            tunnel: "milliseconds to wait\nafter NOTE trigger" -> [w325]
            tunnel: w316 -> [w330]
            tunnel: w313 -> [w327]
            frame #0 {
              n164 = Wait (ms)(milliseconds to wait=w318) -> ()  [unwired: 1 out]
            }
            frame #1 {
              # "STOP INTAKE"
              n165 = Unbundle By Name(w323) -> ("INTAKE ref"=w320:T5)
              n166 = call <vilib>:"SPARK Set Output Advanced.vi"("Control Mode"=Spark_MAX_Control_Type."Percent VBus", "Setpoint"=0.0, "MotorControlDevRef"=w320) -> ("error out"=w324:errorcluster)  [unwired: 7 in, 1 out]
            }
            frame #2 {
              # "DELAY"
              n167 = Wait (ms)(milliseconds to wait=w325) -> ()  [unwired: 1 out]
            }
            frame #3 {
              # "STOP LOADER"
              n168 = Unbundle By Name(w327) -> ("LOADER ref"=w331:T5)
              n169 = call <vilib>:"SPARK Set Output Advanced.vi"("error in (no error)"=w330, "Control Mode"=Spark_MAX_Control_Type."Percent VBus", "Setpoint"=0.0, "MotorControlDevRef"=w331) -> ()  [unwired: 6 in, 2 out]
            }
          }
          n170 = in-place {
            in-place-border: [ctrl_INTAKE_STATES."STANDBY" ("INTAKE STATE 2")] -> w315
            in-place-border: ["shutting down" ("value")] -> w314
          }
        }
      }
    }
    n171 = in-place {
      n172 = case shown="False" "reload global values" {
        tunnel: "LOADER max/min" -> [w208 _]
        tunnel: "LOADER speeds" -> [w207 _]
        tunnel: "SHOOTER speeds" -> [w206 _]
        tunnel: "INTAKE speeds" -> [w205 _]
        frame False {
          n173 = case shown="True" "WRITE to global" {
            tunnel: w208 -> [_ w213]
            tunnel: w207 -> [_ w212]
            tunnel: w206 -> [_ w211]
            tunnel: w205 -> [_ w210]
            frame False {
            }
            frame True {
              n174 = global write "Global INIT.vi" "INTAKE speeds"(w210) -> ()
              n175 = global write "Global INIT.vi" "SHOOTER speeds"(w211) -> ()
              n176 = global write "Global INIT.vi" "LOADER speeds"(w212) -> ()
              n177 = global write "Global INIT.vi" "LOADER max/min"(w213) -> ()
              n178 = local write "WRITE to global"(FALSE ("WRITE to global")) -> ()
            }
          }
        }
        frame True {
          n179 = global read "Global INIT.vi" "INTAKE speeds"() -> (w218:T1)
          n180 = global read "Global INIT.vi" "SHOOTER speeds"() -> (w217:T2)
          n181 = global read "Global INIT.vi" "LOADER speeds"() -> (w216:T1)
          n182 = global read "Global INIT.vi" "LOADER max/min"() -> (w215:T1)
          n183 = local write "reload global values"(FALSE ("reload global values")) -> ()
          n184 = local write "INTAKE speeds"(w218) -> ()
          n185 = local write "SHOOTER speeds"(w217) -> ()
          n186 = local write "LOADER speeds"(w216) -> ()
          n187 = local write "LOADER max/min"(w215) -> ()
        }
      }
    }
    n188 = local write "INTAKE STATUS"(w194) -> ()
  }
